vi "新版温升-不控制电流-TDMS-热电偶-20210323.vi"(0 "file path (dialog if empty)":path caption="文件路径 （空时为对话框）", 1 "总记录时间（H）":dbl, 5 "温度读取地址":refnum<visa-resource-name>="GPIB0::16::INSTR", 9 "样品名称":string, 11 "error in (no error)":errorcluster caption="错误输入（无错误）", 12 "延迟时间（s）":dbl) -> (2 "通道":string[][](array[string]) caption="所有行", 3 "测量通道":string[][](table)=[["110", "侧壁"], ["109", "水泥"], ["108", "底面"], ["107", "端子A"], ["106", "端子B"], ["105", "环境温度"]], 6 "温度情况":string[][](table), 13 "温度曲线":waveform(dbl)[](graph), 14 "数据":waveform(dbl)[](array[waveform]), 15 "错误输出":errorcluster)   [LabVIEW 2021]
uses:
  2700/2700.lvclass
  6510/6510.lvclass
  <vilib>/Utility/file.llb/Read Delimited Spreadsheet (string).vi
  <vilib>/regexp/Match Regular Expression.xnode
  DMM/DMM.lvclass
panel:
  in  "选项卡控件":enum32{"通道配置", "温度曲线"}(tab)
  # "时间"
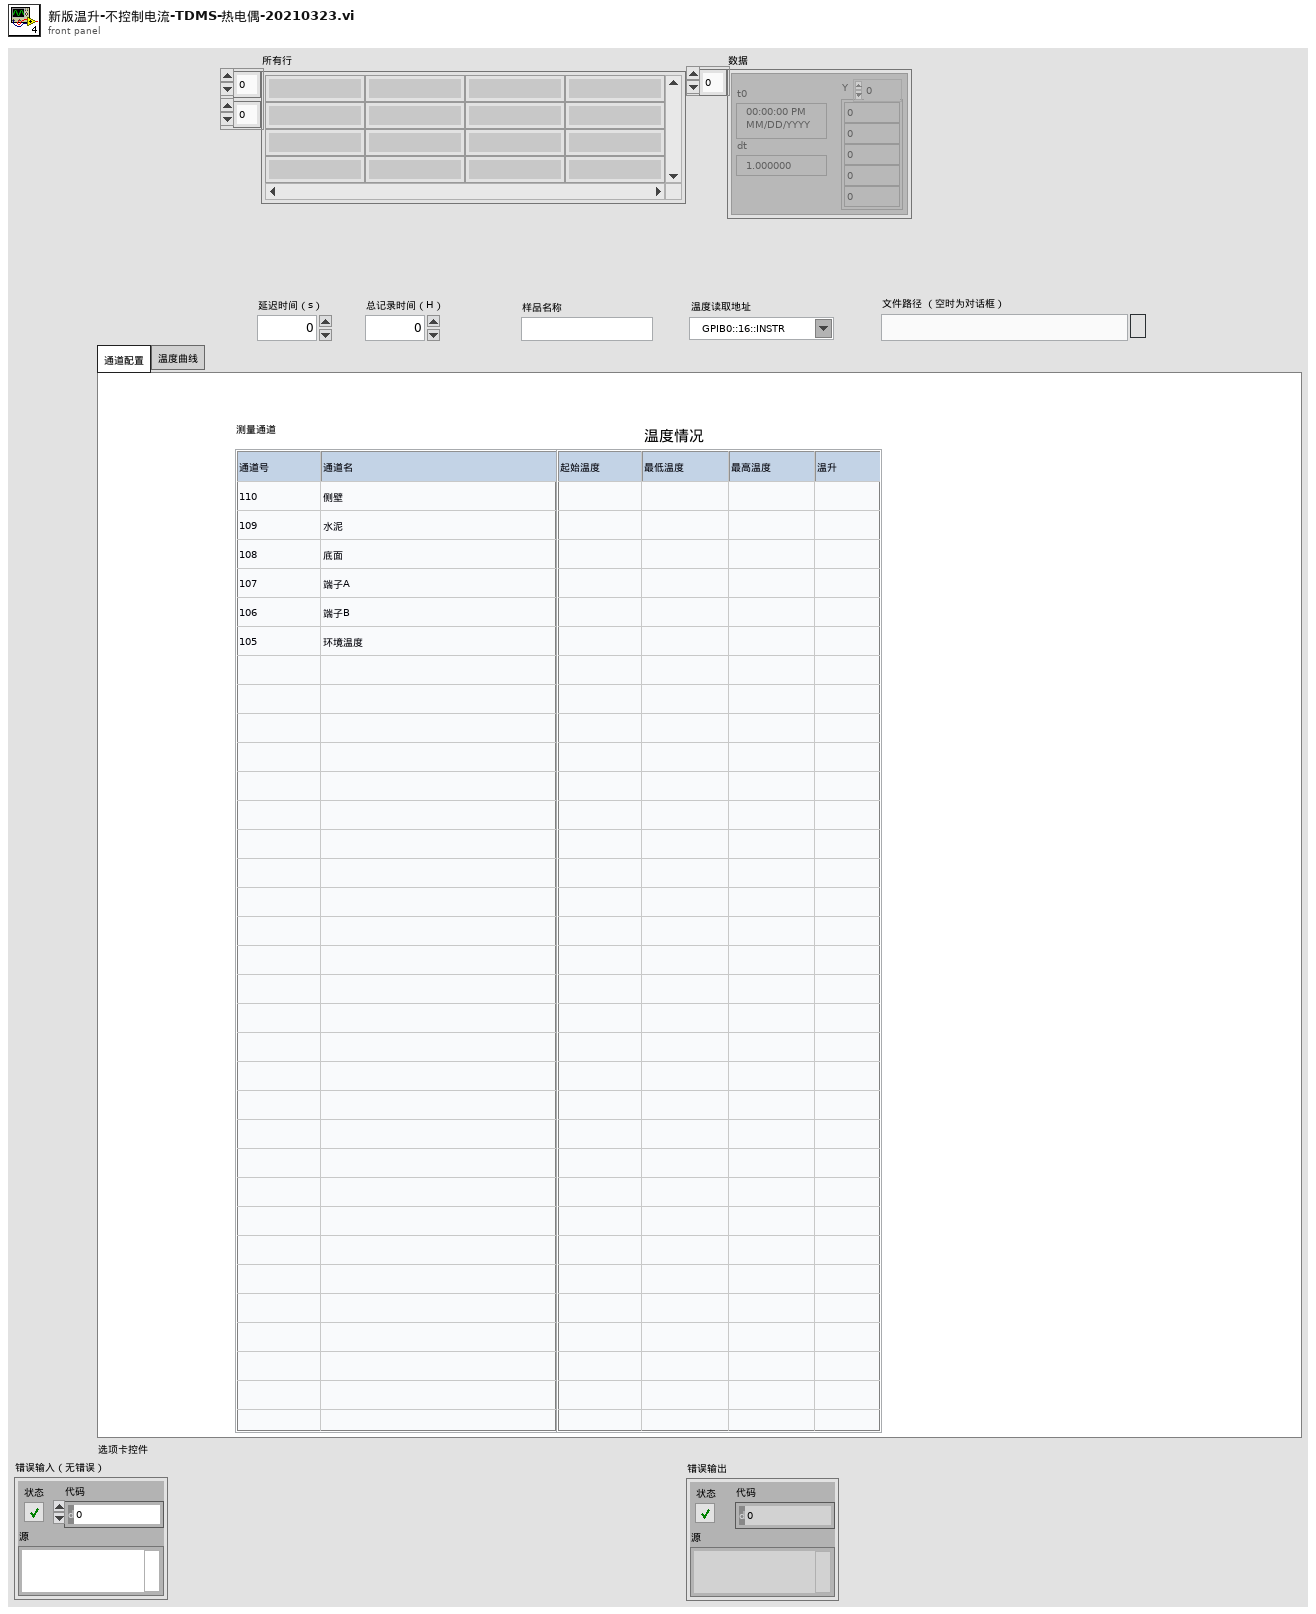
[diagram p1: front panel]
types:
  T1 = enum16{"open", "open or create", "create or replace", "create", "open (read-only)"}
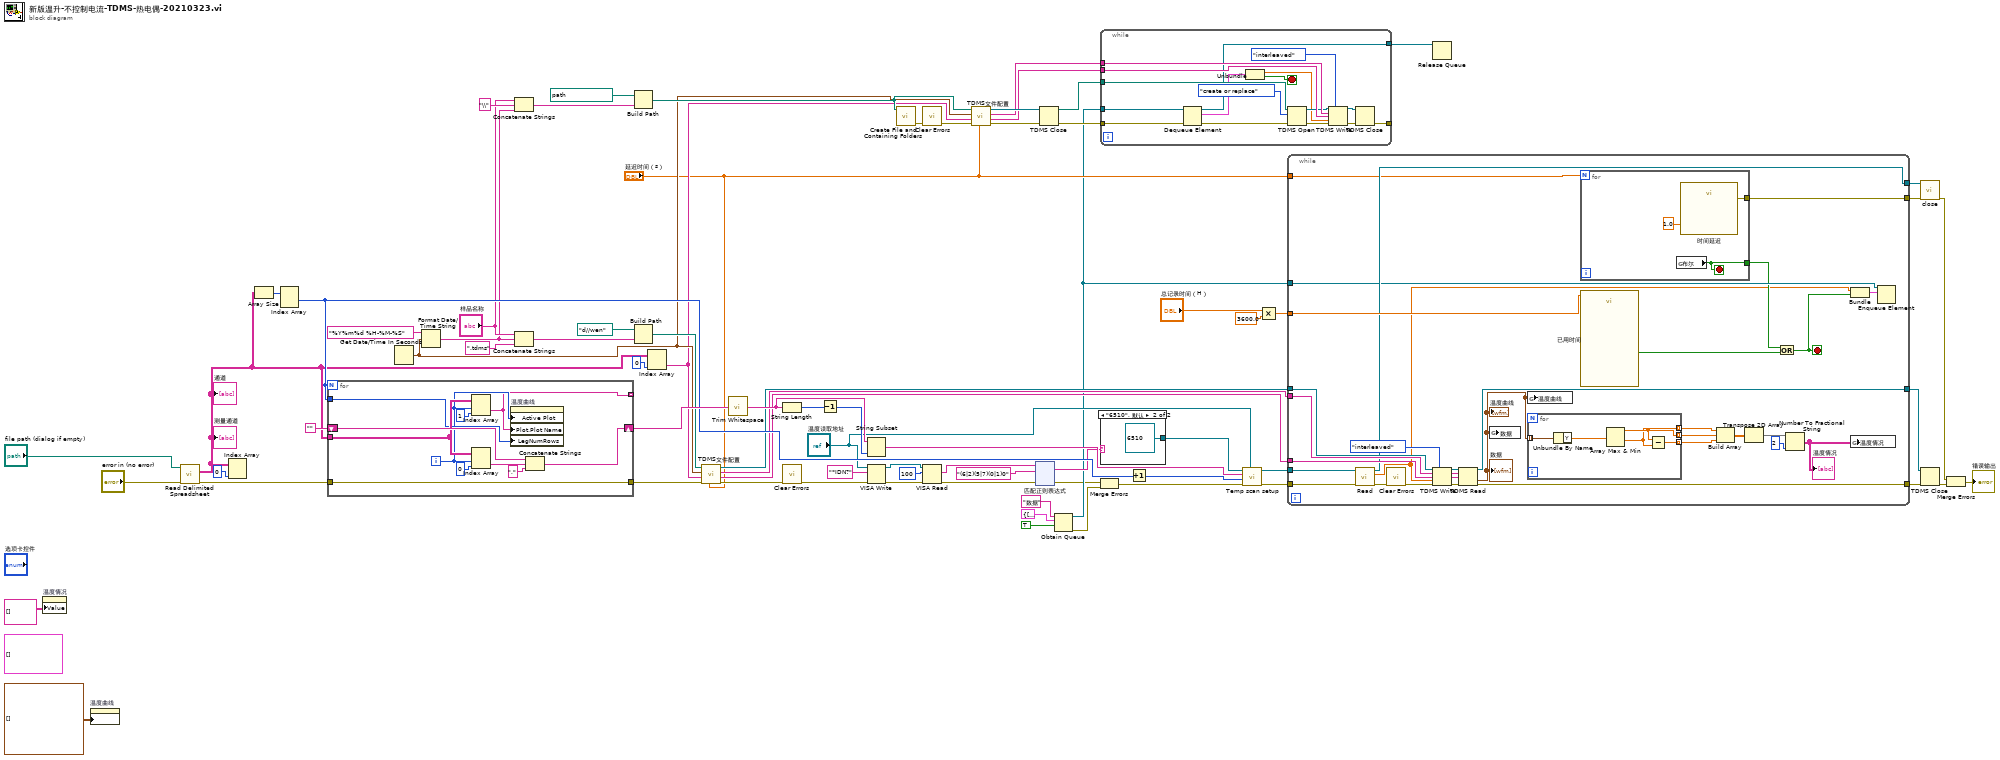
[diagram p0: block diagram]
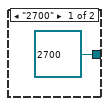
[diagram p2: hidden frame]
diagram:
  (unwired) cluster{dbl[], dbl[]}[] [] ("温度曲线")
  n1 = property on="温度情况" class="Tbl (严格)"("Value"=string[][] [] ("温度情况")) -> ()  [unwired: 2 in, 2 out]
  n2 = property on="温度曲线" class="WFChart (严格)"("History Data"=waveform(dbl)[][] [] ("历史数据")) -> ()  [unwired: 2 in, 2 out]
  n3 = call-poly <vilib>:"Read Delimited Spreadsheet.vi"("file path (dialog if empty)"="file path (dialog if empty)", "error in (no error)"="error in (no error)") -> ("all rows"=w58:string[][], "error out"=w1:errorcluster)  [unwired: 8 in, 4 out]
  "测量通道" <- w58
  "通道" <- w58
  n4 = Index Array(array=w58, index (col)=0 ("禁用的索引 (列)")) -> ()  [unwired: 1 in, 1 out]
  n5 = Array Size(array=w58) -> (size(s)=w75:i32[])
  n6 = Index Array(array=w75) -> (element #1=w65:i32)  [unwired: 2 in, 1 out]
  n7 = for {
    N: w65 -> [_]
    shift-right: [w85] -> w71
    shift-left: "" -> [w84]
    tunnel: w65 -> [w78]
    tunnel: w58 -> [w81]
    tunnel: [w76] -> _ mode=indexing
    tunnel: w1 -> [w79]
    tunnel: [w79] -> w56
    i -> [w77]
    n8 = Index Array(array=w81, index (row)=w77, index (col)=1 ("禁用的索引 (行)")) -> (element=w76:string)
    n9 = Index Array(array=w81, index (row)=w77, index (col)=0 ("禁用的索引 (列)")) -> (element=w80:string)
    n10 = property on="温度曲线" class="WFChart (严格)"("Active Plot"=w77, "Plot.Plot Name"=w76, "LegNumRows"=w78) -> ()  [unwired: 2 in, 2 out]
    n11 = Concatenate Strings(w84, w80, ",") -> (w85:string)
  }
  n12 = Get Date/Time In Seconds() -> (seconds since 1Jan1904=w16:timestamp)
  n13 = Format Date/Time String(time format string (%c)="%Y%m%d %H-%M-%S" ("时间格式字符串(%c)"), seconds (now)=w16) -> (date/time string=w17:string)  [unwired: 1 in]
  n14 = Concatenate Strings("样品名称", "\\" ("字符串"), w17) -> (w30:string)
  n15 = Concatenate Strings("样品名称", w17, ".tdms") -> (w63:string)
  n16 = Build Path(base path=path "d:/温升试验数据" ("基路径"), name or relative path=w30) -> (appended path=w21:path)
  n17 = Build Path(base path=path "d://wen" ("file path (dialog if empty)"), name or relative path=w63) -> (appended path=w59:path)
  n18 = Index Array(array=w58, index (col)=0 ("禁用的索引 (列)")) -> (element=w15:string[])  [unwired: 1 in]
  n19 = call "TDMS文件配置.vi"("时间间隔（s）"="延迟时间（s）", "错误输入（无错误）"=w56, "通道列表"=w15, "时间标识输入控件"=w16, "文件路径"=w59) -> ("error out"=w55:errorcluster, "通道列表"=w52:string[], "group name out"=w53:string, "tdms file out"=w54:refnum<k34>)  [unwired: 3 in]
  n20 = call <vilib>:"Trim Whitespace.vi"("string"=w71) -> ("trimmed string"=w70:string)  [unwired: 1 in]
  n21 = String Length(string=w70) -> (length=w73:i32)
  n22 = call <vilib>:"Clear Errors.vi"("error in (no error)"=w55) -> ("error out"=w37:errorcluster)  [unwired: 5 in, 1 out]
  n23 = Decrement(x=w73) -> (x-1=w72:i32)
  n24 = String Subset(string=w70, length (rest)=w72) -> (substring=w47:string)  [unwired: 1 in]
  n25 = VISA Write(VISA resource name="温度读取地址", write buffer="*IDN?" ("写入缓冲区"), error in (no error)=w37) -> (VISA resource name out=w43:refnum<visa-resource-name>, error out=w44:errorcluster)  [unwired: 1 out]
  n26 = call <vilib>:"Create File and Containing Folders.vi"("file path"=w21) -> ("error out"=w22:errorcluster)  [unwired: 9 in, 1 out]
  n27 = call <vilib>:"Clear Errors.vi"("error in (no error)"=w22) -> ("error out"=w20:errorcluster)  [unwired: 5 in, 1 out]
  n28 = VISA Read(VISA resource name=w43, byte count=u32 100 ("字节总数"), error in (no error)=w44) -> (read buffer=w40:string, error out=w39:errorcluster)  [unwired: 2 out]
  n29 = call "TDMS文件配置.vi"("时间间隔（s）"="延迟时间（s）", "错误输入（无错误）"=w20, "通道列表"=w15, "时间标识输入控件"=w16, "文件路径"=w21) -> ("error out"=w28:errorcluster, "通道列表"=w23:string[], "group name out"=w24:string, "tdms file out"=w27:refnum<k34>)  [unwired: 3 in]
  n30 = xnode "匹配正则表达式"("输入字符串"=w40, "正则表达式"="(6|2)(5|7)(0|1)0", "错误输入"=w39) -> ("所有匹配"=w38:string, "错误输出"=w8:errorcluster)  [unwired: 3 in, 3 out]
  n31 = TDMS Close(8:w28, 11:w27) -> (0:w26:errorcluster, 3:w25:path)
  n32 = Obtain Queue(name (unnamed)="数据" ("名称（未命名）"), element data type=cluster{"数组":dbl[], bool} {"数组"=[40.5266151, 40.9824181, 39.4802208], FALSE}, create if not found? (T)=TRUE ("如未找到则创建？(T)")) -> (queue out=w10:refnum<queue>, error out=w7:errorcluster)  [unwired: 2 in, 1 out]
  n33 = while {
    tunnel: w26 -> [w91]
    tunnel: w25 -> [w103]
    tunnel: w24 -> [w102]
    tunnel: w23 -> [w101]
    tunnel: w10 -> [w94]
    tunnel: [w93] -> w19
    tunnel: [w88] -> _
    stop <- w87 stop-if-true
    n34 = Dequeue Element(queue=w94, error in (no error)=w91) -> (queue out=w93:refnum<queue>, element=w90:cluster{"数组":dbl[], bool}, error out=w95:errorcluster)  [unwired: 1 in, 1 out]
    n35 = Unbundle(w90) -> ("数组"=w89:dbl[], w87:bool)
    n36 = TDMS Open(8:w95, 10:T1."create or replace" ("操作(0:open)"), 11:w103) -> (0:w100:errorcluster, 3:w99:refnum<k34>)  [unwired: 4 in]
    n37 = TDMS Write(0:w99, 1:enum16{"decimated", "interleaved"}."interleaved" ("数据布局（0:降采样）"), 5:w102, 7:w101, 9:w89, 11:w100) -> (4:w96:refnum<k34>, 15:w97:errorcluster)  [unwired: 2 out]
    n38 = TDMS Close(8:w97, 11:w96) -> (0:w88:errorcluster)  [unwired: 1 out]
  }
  n39 = case shown="\"6510\", 默认" w38 {
    tunnel: [refnum<class "2700.lvclass"> refnum ("2700.lvclass") refnum<class "6510.lvclass"> refnum ("6510.lvclass")] -> w35
    frame "2700" {
    }
    frame "6510", Default {
    }
  }
  n40 = Merge Errors(w8, w7) -> (w6:errorcluster)
  n41 = Increment(x=w65) -> (x+1=w48:i32)
  n42 = call-dynamic "Temp scan setup.vi"("VISA资源名称"="温度读取地址", "error in (no error)"=w6, "数值"=w48, "字符串"=w47, "DMM 输入"=w35) -> ("error out"=w46:errorcluster, "DMM 输出"=w34:refnum<class "DMM.lvclass">)  [unwired: 5 in]
  n43 = Multiply(x="总记录时间（H）", y=3600.0) -> (x*y=w67:dbl)
  n44 = while {
    tunnel: w46 -> [w118]
    tunnel: [w117] -> w33
    tunnel: w67 -> [w137]
    tunnel: [w120] -> w60
    tunnel: w54 -> [w128]
    tunnel: w53 -> [w127]
    tunnel: w52 -> [w126]
    tunnel: [w121] -> w51
    tunnel: "延迟时间（s）" -> [w115]
    tunnel: w34 -> [w119]
    tunnel: w10 -> [w116]
    tunnel: [w111] -> w9
    stop <- w113 stop-if-true
    n45 = call-dynamic "Read.vi"("error in (no error)"=w118, "DMM 输入"=w119) -> ("error out"=w108:errorcluster, "数组"=w106:dbl[], "DMM 输出"=w117:refnum<class "DMM.lvclass">)  [unwired: 7 in]
    n46 = call <vilib>:"Clear Errors.vi"("error in (no error)"=w108) -> ("error out"=w107:errorcluster)  [unwired: 5 in, 1 out]
    n47 = TDMS Write(0:w128, 1:enum16{"decimated", "interleaved"}."interleaved" ("数据布局（0:降采样）"), 5:w127, 7:w126, 9:w106, 11:w107) -> (4:w125:refnum<k34>, 6:w124:string, 8:w123:string[], 15:w122:errorcluster)
    n48 = TDMS Read(0:w125, 5:w124, 7:w123, 11:w122) -> (4:w120:refnum<k34>, 10:w109:waveform(dbl)[], 15:w121:errorcluster)  [unwired: 4 in, 3 out]
    "温度曲线" <- w109
    "数据" <- w109
    n49 = global write "数据传输.vi" "数据"(w109) -> ()
    n50 = global write "数据传输.vi" "温度曲线"(w109) -> ()
    n51 = for {
      tunnel: w109 -> [w142] mode=indexing
      tunnel: [w145] -> w135 mode=indexing
      tunnel: [w144] -> w134 mode=indexing
      tunnel: [w143] -> w133 mode=indexing
      n52 = Unbundle By Name(w142) -> ("Y"=w141:dbl[])
      n53 = Array Max & Min(array=w141) -> (max value=w145:dbl, min value=w144:dbl)  [unwired: 2 out]
      n54 = Subtract(x=w145, y=w144) -> (x-y=w143:dbl)
    }
    n55 = for {
      N: w115 -> [_]
      tunnel: [w138] -> w114
      tunnel: [w139] -> w111
      stop <- w138 stop-if-true
      n56 = global read "数据传输.vi" "布尔"() -> (w138:bool)
      n57 = call "时间延迟"("Delay Time (s)"=1.0) -> ("error out"=w139:errorcluster)  [unwired: 10 in]
    }
    n58 = call "已用时间"("Time Target (s)"=w137) -> ("Time has Elapsed"=w136:bool)  [unwired: 11 in, 7 out]
    n59 = Build Array(w134, w135, w133) -> (w132:dbl[][])
    n60 = Transpose 2D Array(2D array=w132) -> (transposed array=w131:dbl[][])
    n61 = Or(x=w114, y=w136) -> (x .or. y?=w113:bool)
    n62 = Number To Fractional String(number=w131, precision (6)=i16 2 ("精度(6)")) -> (F-format string=w110:string[][])  [unwired: 2 in]
    "温度情况" <- w110
    n63 = Bundle("数组"=w106, w113) -> (w112:cluster{"数组":dbl[], bool})  [unwired: 1 in]
    n64 = global write "数据传输.vi" "温度情况"(w110) -> ()
    n65 = Enqueue Element(queue=w116, element=w112) -> ()  [unwired: 2 in, 3 out]
  }
  n66 = Release Queue(queue=w19) -> ()  [unwired: 2 in, 3 out]
  n67 = call-dynamic "close.vi"("error in (no error)"=w9, "DMM 输入"=w33) -> ("error out"=w4:errorcluster)  [unwired: 8 in, 1 out]
  n68 = TDMS Close(8:w51, 11:w60) -> (0:w3:errorcluster)  [unwired: 1 out]
  n69 = Merge Errors(w4, w3) -> (→"错误输出":errorcluster)
